vi "myRIO_BRig_Host_TCP_parseCmd_selectResponse__subunit2.vi"(0 "input_idxReward":i32, 1 "input_arrayReward":i32[][](array[numeric]), 2 "input_idxWrong":i32, 3 "input_arrayWrong":i32[][](array[numeric]), 4 "input_idxTimeout":i32, 5 "input_arrayTimeout":i32[][](array[numeric]), 6 "input_response":i32, 8 "input_L/R":i32, 10 "input_countTrial":i32) -> (14 "output_idxReward":i32, 15 "output_arrayReward":i32[][](array[numeric]), 16 "output_idxWrong":i32, 17 "output_arrayWrong":i32[][](array[numeric]), 18 "output_idxTimeout":i32, 19 "output_arrayTimeout":i32[][](array[numeric]))   [LabVIEW 2014]
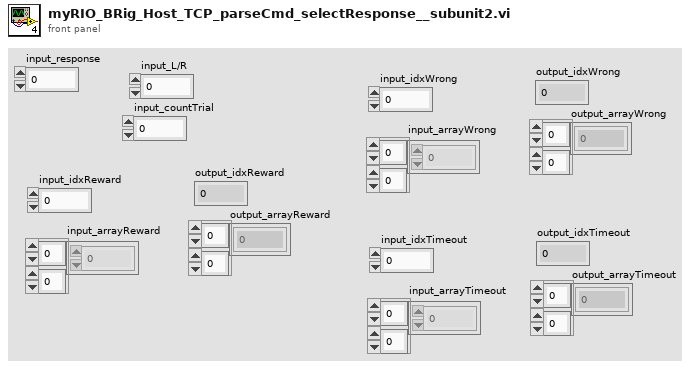
[diagram p1: front panel]
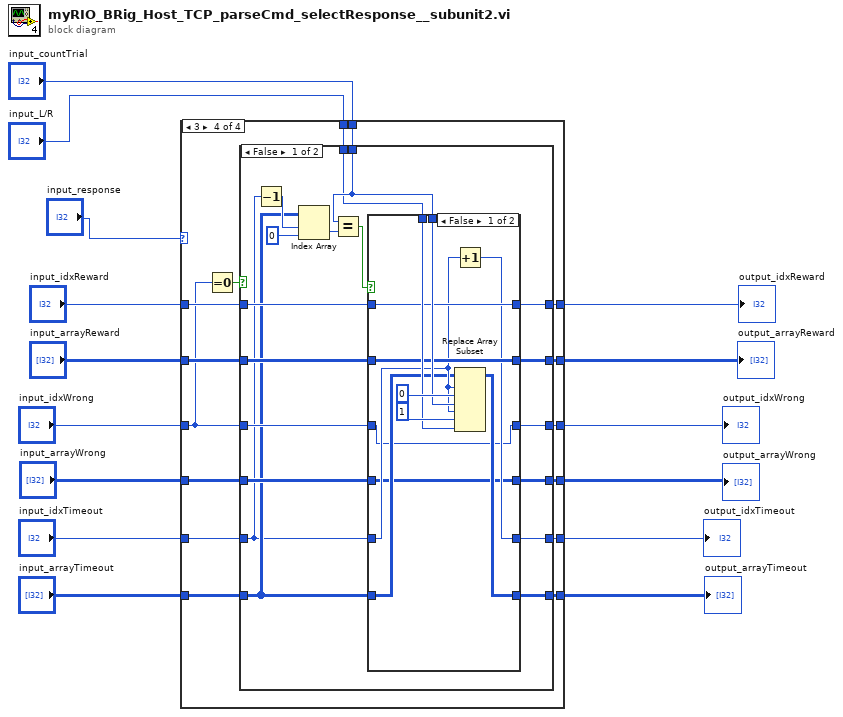
[diagram p0: block diagram]
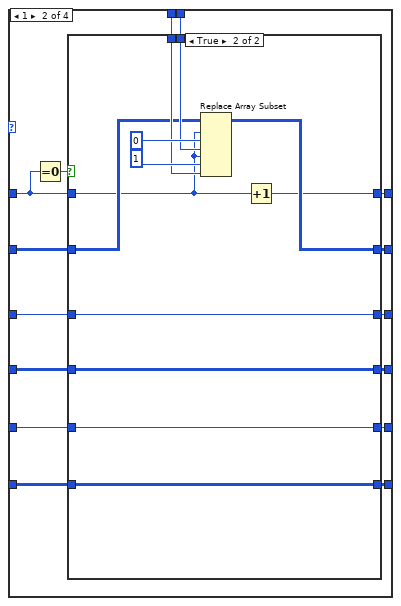
[diagram p3: hidden frame]
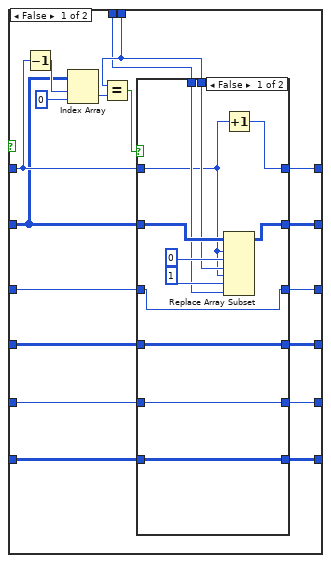
[diagram p4: hidden frame]
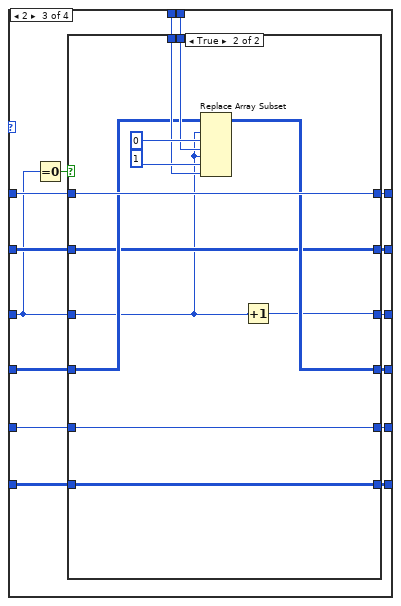
[diagram p6: hidden frame]
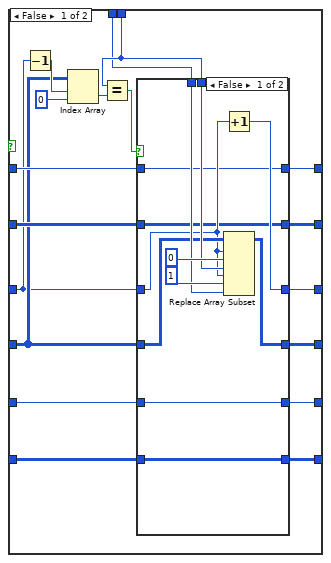
[diagram p7: hidden frame]
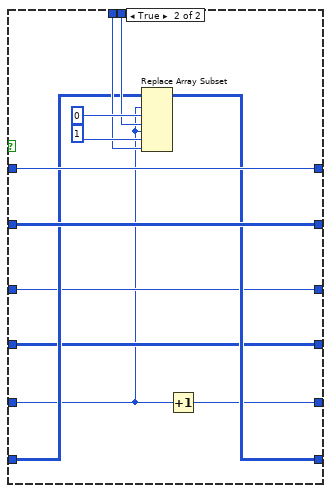
[diagram p10: hidden frame]
diagram:
  n1 = case shown="3" "input_response" {
    tunnel: "input_idxReward" -> [w21 w34 w97 w160]
    tunnel: "input_arrayReward" -> [w20 w35 w98 w161]
    tunnel: "input_countTrial" -> [_ w33 w96 w159]
    tunnel: "input_L/R" -> [_ w32 w95 w158]
    tunnel: [w20 w31 w94 w157] -> w10
    tunnel: [w21 w30 w93 w156] -> w9
    tunnel: "input_idxWrong" -> [w19 w29 w85 w148]
    tunnel: "input_arrayWrong" -> [w18 w27 w91 w154]
    tunnel: [w19 w28 w92 w155] -> w6
    tunnel: [w18 w26 w90 w153] -> w5
    tunnel: "input_idxTimeout" -> [w17 w25 w89 w152]
    tunnel: [w17 w24 w88 w151] -> w3
    tunnel: "input_arrayTimeout" -> [w16 w23 w87 w150]
    tunnel: [w16 w22 w86 w149] -> w1
    frame 0, Default {
    }
    frame 1 {
      n2 = Equal To 0?(x=w34) -> (x = 0?=w36:bool)
      n3 = case shown="True" w36 {
        tunnel: w35 -> [w47 w79]
        tunnel: w34 -> [w49 w74]
        tunnel: w33 -> [w46 w82]
        tunnel: w32 -> [w45 w81]
        tunnel: [w48 w80] -> w31
        tunnel: [w50 w73] -> w30
        tunnel: w29 -> [w44 w78]
        tunnel: [w43 w78] -> w28
        tunnel: w27 -> [w42 w77]
        tunnel: [w41 w77] -> w26
        tunnel: w25 -> [w40 w76]
        tunnel: [w39 w76] -> w24
        tunnel: w23 -> [w38 w75]
        tunnel: [w37 w75] -> w22
        frame False {
          n4 = Decrement(x=w49) -> (x-1=w54:i32)
          n5 = Index Array(array=w47, index (row)=w54, index (col)=0 ("disabled index (col)")) -> (element=w51:i32)
          n6 = Equal?(x=w46, y=w51) -> (x = y?=w53:bool)
          n7 = case shown="False" w53 {
            tunnel: [w59 w72] -> w50
            tunnel: w49 -> [w60 w72]
            tunnel: [w64 w71] -> w48
            tunnel: w47 -> [w63 w71]
            tunnel: w46 -> [w62 _]
            tunnel: w45 -> [w61 _]
            tunnel: w44 -> [w58 w70]
            tunnel: [w58 w70] -> w43
            tunnel: w42 -> [w57 w69]
            tunnel: [w57 w69] -> w41
            tunnel: w40 -> [w56 w68]
            tunnel: [w56 w68] -> w39
            tunnel: w38 -> [w55 w67]
            tunnel: [w55 w67] -> w37
            frame False {
              n8 = Increment(x=w60) -> (x+1=w59:i32)
              n9 = Replace Array Subset(array=w63, new element #1=w62, index (row) #1=w60, index (col) #1=0 ("new element/subarray"), new element #2=w61, index (row) #2=w60, index (col) #2=1 ("new element/subarray")) -> (w64:i32[][])
            }
            frame True {
            }
          }
        }
        frame True {
          n10 = Replace Array Subset(array=w79, new element #1=w82, index (row) #1=w74, index (col) #1=0 ("disabled index (col)"), new element #2=w81, index (row) #2=w74, index (col) #2=1 ("disabled index (col)")) -> (w80:i32[][])
          n11 = Increment(x=w74) -> (x+1=w73:i32)
        }
      }
    }
    frame 2 {
      n12 = Equal To 0?(x=w85) -> (x = 0?=w99:bool)
      n13 = case shown="True" w99 {
        tunnel: w98 -> [w110 w138]
        tunnel: w97 -> [w112 w143]
        tunnel: w96 -> [w109 w145]
        tunnel: w95 -> [w108 w144]
        tunnel: [w111 w138] -> w94
        tunnel: [w113 w143] -> w93
        tunnel: w85 -> [w100 w137]
        tunnel: [w107 w136] -> w92
        tunnel: w91 -> [w101 w140]
        tunnel: [w106 w139] -> w90
        tunnel: w89 -> [w105 w142]
        tunnel: [w104 w142] -> w88
        tunnel: w87 -> [w103 w141]
        tunnel: [w102 w141] -> w86
        frame False {
          n14 = Decrement(x=w100) -> (x-1=w117:i32)
          n15 = Index Array(array=w101, index (row)=w117, index (col)=0 ("disabled index (col)")) -> (element=w114:i32)
          n16 = Equal?(x=w109, y=w114) -> (x = y?=w116:bool)
          n17 = case shown="False" w116 {
            tunnel: [w119 w135] -> w113
            tunnel: w112 -> [w119 w135]
            tunnel: [w118 w134] -> w111
            tunnel: w110 -> [w118 w134]
            tunnel: w109 -> [w127 _]
            tunnel: w108 -> [w126 _]
            tunnel: w100 -> [w121 w133]
            tunnel: [w120 w133] -> w107
            tunnel: w101 -> [w123 w132]
            tunnel: [w122 w132] -> w106
            tunnel: w105 -> [w125 w131]
            tunnel: [w125 w131] -> w104
            tunnel: w103 -> [w124 w130]
            tunnel: [w124 w130] -> w102
            frame False {
              n18 = Increment(x=w121) -> (x+1=w120:i32)
              n19 = Replace Array Subset(array=w123, new element #1=w127, index (row) #1=w121, index (col) #1=0 ("new element/subarray"), new element #2=w126, index (row) #2=w121, index (col) #2=1 ("new element/subarray")) -> (w122:i32[][])
            }
            frame True {
            }
          }
        }
        frame True {
          n20 = Replace Array Subset(array=w140, new element #1=w145, index (row) #1=w137, index (col) #1=0 ("disabled index (col)"), new element #2=w144, index (row) #2=w137, index (col) #2=1 ("disabled index (col)")) -> (w139:i32[][])
          n21 = Increment(x=w137) -> (x+1=w136:i32)
        }
      }
    }
    frame 3 {
      n22 = Equal To 0?(x=w148) -> (x = 0?=w162:bool)
      n23 = case shown="False" w162 {
        tunnel: w161 -> [w173 w205]
        tunnel: w160 -> [w175 w206]
        tunnel: w159 -> [w172 w208]
        tunnel: w158 -> [w171 w207]
        tunnel: [w174 w205] -> w157
        tunnel: [w176 w206] -> w156
        tunnel: w148 -> [w165 w201]
        tunnel: [w170 w201] -> w155
        tunnel: w154 -> [w166 w202]
        tunnel: [w169 w202] -> w153
        tunnel: w152 -> [w163 w200]
        tunnel: [w168 w199] -> w151
        tunnel: w150 -> [w164 w204]
        tunnel: [w167 w203] -> w149
        frame False {
          n24 = Decrement(x=w163) -> (x-1=w180:i32)
          n25 = Index Array(array=w164, index (row)=w180, index (col)=0 ("disabled index (col)")) -> (element=w177:i32)
          n26 = Equal?(x=w172, y=w177) -> (x = y?=w179:bool)
          n27 = case shown="False" w179 {
            tunnel: [w188 w198] -> w176
            tunnel: w175 -> [w188 w198]
            tunnel: [w187 w197] -> w174
            tunnel: w173 -> [w187 w197]
            tunnel: w172 -> [w190 _]
            tunnel: w171 -> [w189 _]
            tunnel: w165 -> [w181 w196]
            tunnel: [w181 w196] -> w170
            tunnel: w166 -> [w182 w195]
            tunnel: [w182 w195] -> w169
            tunnel: w163 -> [w186 w194]
            tunnel: [w184 w194] -> w168
            tunnel: w164 -> [w185 w193]
            tunnel: [w183 w193] -> w167
            frame False {
              n28 = Increment(x=w186) -> (x+1=w184:i32)
              n29 = Replace Array Subset(array=w185, new element #1=w190, index (row) #1=w186, index (col) #1=0 ("new element/subarray"), new element #2=w189, index (row) #2=w186, index (col) #2=1 ("new element/subarray")) -> (w183:i32[][])
            }
            frame True {
            }
          }
        }
        frame True {
          n30 = Replace Array Subset(array=w204, new element #1=w208, index (row) #1=w200, index (col) #1=0 ("disabled index (col)"), new element #2=w207, index (row) #2=w200, index (col) #2=1 ("disabled index (col)")) -> (w203:i32[][])
          n31 = Increment(x=w200) -> (x+1=w199:i32)
        }
      }
    }
  }
  "output_idxReward" <- w9
  "output_arrayReward" <- w10
  "output_idxWrong" <- w6
  "output_arrayWrong" <- w5
  "output_idxTimeout" <- w3
  "output_arrayTimeout" <- w1
